vi "create.events.vi"(8 "error in (no error)":errorcluster, 11 "EventDaemon in":refnum<class "TemplateDaemon.lvclass">) -> (0 "error out":errorcluster, 3 "EventDaemon out":refnum<class "TemplateDaemon.lvclass">)   [LabVIEW 2024, in "TemplateDaemon.lvclass"]
doc: "Create all event-based messaging."
uses:
  TemplateDaemon.lvclass
  TemplateDaemon.lvclass/TemplateDaemon.ctl
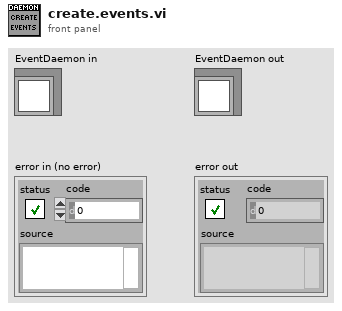
[diagram p1: front panel]
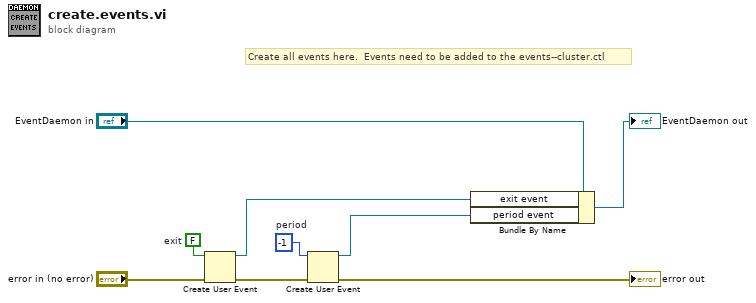
[diagram p0: block diagram]
diagram:
  w4 = -1  # period
  w7 = FALSE  # exit
  # "Create all events here.  Events need to be added to the events--cluster.ctl"
  n1 = Create User Event(user event datatype=w7, error in="error in (no error)") -> (user event=w6:refnum<user-event>, error out=w3:errorcluster)
  n2 = Create User Event(user event datatype=w4, error in=w3) -> (user event=w1:refnum<user-event>, error out=→"error out":errorcluster)
  n3 = Bundle By Name(cluster="EventDaemon in", "exit event"=w6, "period event"=w1) -> (→"EventDaemon out":refnum<class "TemplateDaemon.lvclass">)
